vi "Robot Control.vi"() -> ()   [LabVIEW 2022 SP3]
uses:
  <vilib>/ImagingLab/Denso Robotics Library/_Private/Controls/drl_Motion parameters.ctl
  <vilib>/ImagingLab/Denso Robotics Library/_Private/Controls/drl_Interpolation.ctl
  <vilib>/ImagingLab/Denso Robotics Library/_Private/Controls/drl_Pass motion.ctl
  <vilib>/ImagingLab/Denso Robotics Library/_Private/Controls/drl_Move option.ctl
  <vilib>/ImagingLab/Denso Robotics Library/_Private/Controls/drl_Robot Coordinates.ctl
  <vilib>/ImagingLab/Denso Robotics Library/_Private/Controls/drl_Variable J.ctl
  <vilib>/ImagingLab/Denso Robotics Library/_Private/Controls/drl_Variable T.ctl
  <vilib>/ImagingLab/Denso Robotics Library/_Private/Controls/drl_TOOL.ctl
  <vilib>/ImagingLab/Denso Robotics Library/_Private/Controls/drl_arch_parameters.ctl
  <vilib>/ImagingLab/Denso Robotics Library/_Private/Controls/drl_Position Type.ctl
  <vilib>/ImagingLab/Denso Robotics Library/_Private/Controls/drl_Open Data.ctl
  <vilib>/ImagingLab/Denso Robotics Library/_Private/Controls/drl_Controller_IP Address.ctl
  <vilib>/ImagingLab/Denso Robotics Library/_Private/Controls/drl_Robot type.ctl
  <vilib>/ImagingLab/Denso Robotics Library/_Private/Controls/drl_controller_type.ctl
  <vilib>/ImagingLab/Denso Robotics Library/_Private/Controls/drl_Robot Session.ctl
  <vilib>/ImagingLab/Denso Robotics Library/_Private/Controls/drl_RobSlave actions.ctl
  <vilib>/ImagingLab/Denso Robotics Library/_Private/Controls/drl_Robot Motor status.ctl
  <vilib>/ImagingLab/Denso Robotics Library/_Private/Controls/drl_Get_Set.ctl
  <vilib>/Utility/error.llb/DialogType.ctl
  <vilib>/ImagingLab/Denso Robotics Library/_Public/SubVIs/drl_Get_Robot Position_P.vi
  <vilib>/ImagingLab/Denso Robotics Library/_Public/SubVIs/drl_Get_Robot Angle_J.vi
  <vilib>/ImagingLab/Denso Robotics Library/_Public/SubVIs/drl_Get_Robot Trans_T.vi
  <vilib>/ImagingLab/Denso Robotics Library/_Public/SubVIs/drl_Robot Move_CARTESIAN.vi
  <vilib>/ImagingLab/Denso Robotics Library/_Public/SubVIs/drl_Robot Move_JOINT.vi
  <vilib>/ImagingLab/Denso Robotics Library/_Public/SubVIs/drl_Set_Get Variable_P.vi
  <vilib>/ImagingLab/Denso Robotics Library/DensoRoboticsLibrary.lvlib
panel:
  in  "Main Tab Control":T1(tab)
  in  "Move Tab Control":enum32{"Cartesian", "Joint"}(tab)
  in  "Move to position C":bool
  in  "robot coordinates C":T2 {"X" format="%.4f"; "Y" format="%.4f"; "Z" format="%.4f"; "Rx" format="%.4f"; "Ry" format="%.4f"; "Rz" format="%.4f"}
  in  "motion parameters C":T3
  in  "Load position C":bool
  in  "Move to position J":bool
  in  "motion parameters J":T3
  in  "Load position J":bool
  in  "robot coordinates J":T7 {"Axis 6" format="%.4f"; "Axis 5" format="%.4f"; "Axis 4" format="%.4f"; "Axis 3" format="%.4f"; "Axis 2" format="%.4f"; "Axis 1" format="%.4f"}
  in  "Set tool active":bool
  in  "Set tool params":bool
  in  "Tool data":T8
  in  "Tool number set":i32
  in  "Active tool":i32
  in  "Tab Control":enum32{"Cart", "Joint"}(tab)
  in  "Drive cart":bool
  out "Velocity start cart":T2 {"X" format="%.4f"; "Y" format="%.4f"; "Z" format="%.4f"; "Rx" format="%.4f"; "Ry" format="%.4f"; "Rz" format="%.4f"}
  out "Current step cart":i32
  in  "velocity motion parameters cart":T3
  in  "Velocity step cart":T2 {"X" format="%.4f"; "Y" format="%.4f"; "Z" format="%.4f"; "Rx" format="%.4f"; "Ry" format="%.4f"; "Rz" format="%.4f"}
  in  "Steps cart":i32
  in  "Drive joint":bool
  out "Velocity start joint":T7 {"Axis 6" format="%.4f"; "Axis 5" format="%.4f"; "Axis 4" format="%.4f"; "Axis 3" format="%.4f"; "Axis 2" format="%.4f"; "Axis 1" format="%.4f"}
  in  "velocity motion parameters joint":T3
  out "Current step joint":i32
  in  "Velocity step joint":T7 {"Axis 6" format="%.4f"; "Axis 5" format="%.4f"; "Axis 4" format="%.4f"; "Axis 3" format="%.4f"; "Axis 2" format="%.4f"; "Axis 1" format="%.4f"}
  in  "Steps joints":i32
  in  "Start arch":bool
  in  "position type":T9
  in  "variable P end":T2 {"X" format="%.4f"; "Y" format="%.4f"; "Z" format="%.4f"; "Rx" format="%.4f"; "Ry" format="%.4f"; "Rz" format="%.4f"}
  in  "arch parameters":T10={"height (mm)"=5, "arch start (mm)"=0, "arch finish (mm)"=0}
  in  "Internal speed":dbl=100.0
  in  "External speed":dbl=10.0
  in  "stop":bool
  out "position T":T11 {"Az" format="%.4f"; "Ay" format="%.4f"; "Ax" format="%.4f"; "Oz" format="%.4f"; "Oy" format="%.4f"; "Ox" format="%.4f"; "Z" format="%.4f"; "Y" format="%.4f"; "X" format="%.4f"}
  out "position J":T7 {"Axis 6" format="%.4f"; "Axis 5" format="%.4f"; "Axis 4" format="%.4f"; "Axis 3" format="%.4f"; "Axis 2" format="%.4f"; "Axis 1" format="%.4f"}
  out "position P":T2 {"X" format="%.4f"; "Y" format="%.4f"; "Z" format="%.4f"; "Rx" format="%.4f"; "Ry" format="%.4f"; "Rz" format="%.4f"}
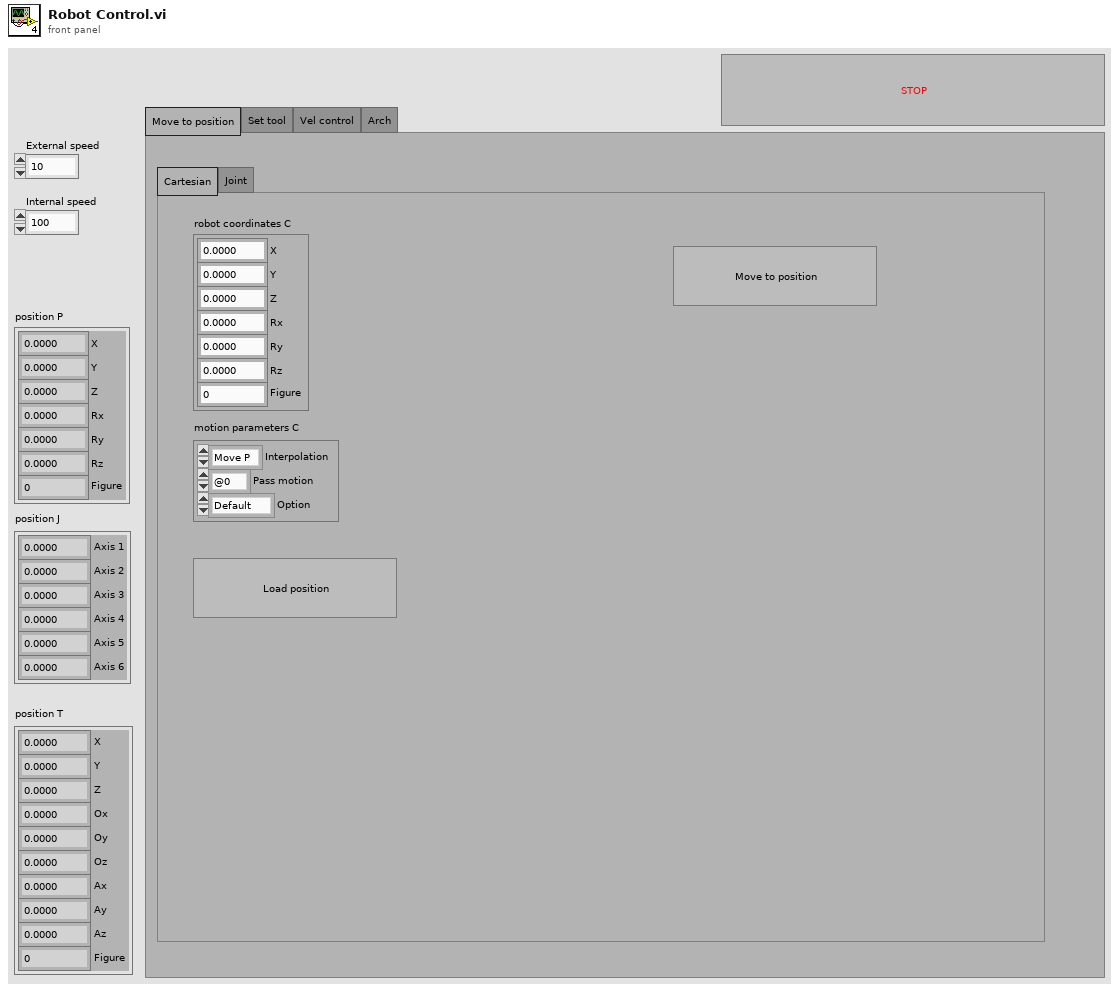
[diagram p1: front panel]
types:
  T1 = enum32{"Move to position", "Set tool", "Vel control", "Arch"}
  T2 = typedef "DensoRoboticsLibrary.lvlib/drl_Robot Coordinates.ctl" = cluster{"X":dbl, "Y":dbl, "Z":dbl, "Rx":dbl, "Ry":dbl, "Rz":dbl, "Figure":dbl}
  T3 = typedef "DensoRoboticsLibrary.lvlib/drl_Motion parameters.ctl" = cluster{"Interpolation":T4, "Pass motion":T5, "Option":T6}
  T4 = typedef "DensoRoboticsLibrary.lvlib/drl_Interpolation.ctl" = enum16{"Move P", "Move L"}
  T5 = typedef "DensoRoboticsLibrary.lvlib/drl_Pass motion.ctl" = enum16{"@0", "@P", "@E"}
  T6 = typedef "DensoRoboticsLibrary.lvlib/drl_Move option.ctl" = enum16{"Default", "Next"}
  T7 = typedef "DensoRoboticsLibrary.lvlib/drl_Variable J.ctl" = cluster{"Axis 1":sgl, "Axis 2":sgl, "Axis 3":sgl, "Axis 4":sgl, "Axis 5":sgl, "Axis 6":sgl}
  T8 = typedef "DensoRoboticsLibrary.lvlib/drl_TOOL.ctl" = cluster{"X":sgl, "Y":sgl, "Z":sgl, "RX":sgl, "RY":sgl, "RZ":sgl}
  T9 = typedef "DensoRoboticsLibrary.lvlib/drl_Position Type.ctl" = enum16{"P", "J", "T"}
  T10 = typedef "DensoRoboticsLibrary.lvlib/drl_arch_parameters.ctl" = cluster{"height (mm)":i32, "arch start (mm)":i32, "arch finish (mm)":i32}
  T11 = typedef "DensoRoboticsLibrary.lvlib/drl_Variable T.ctl" = cluster{"X":sgl, "Y":sgl, "Z":sgl, "Ox":sgl, "Oy":sgl, "Oz":sgl, "Ax":sgl, "Ay":sgl, "Az":sgl, "Figure":sgl}
  T12 = typedef "DensoRoboticsLibrary.lvlib/drl_RobSlave actions.ctl" = enum16{"Start", "Stop"}
  T13 = typedef "DensoRoboticsLibrary.lvlib/drl_Robot Motor status.ctl" = enum16{"Motor OFF", "Motor ON"}
  T14 = typedef "DensoRoboticsLibrary.lvlib/drl_Robot Session.ctl" = string
  T15 = typedef "DensoRoboticsLibrary.lvlib/drl_Open Data.ctl" = cluster{"controller IP address":T16, "robot type":T17, "controller type":T18}
  T16 = typedef "DensoRoboticsLibrary.lvlib/drl_Controller_IP Address.ctl" = string
  T17 = typedef "DensoRoboticsLibrary.lvlib/drl_Robot type.ctl" = enum16{"6 axes", "5 axes", "4 axes"}
  T18 = typedef "DensoRoboticsLibrary.lvlib/drl_controller_type.ctl" = enum16{"RC7", "RC8"}
  T19 = typedef "DensoRoboticsLibrary.lvlib/drl_Get_Set.ctl" = enum16{"Get", "Set"}
  T20 = typedef "DialogType.ctl" = u16
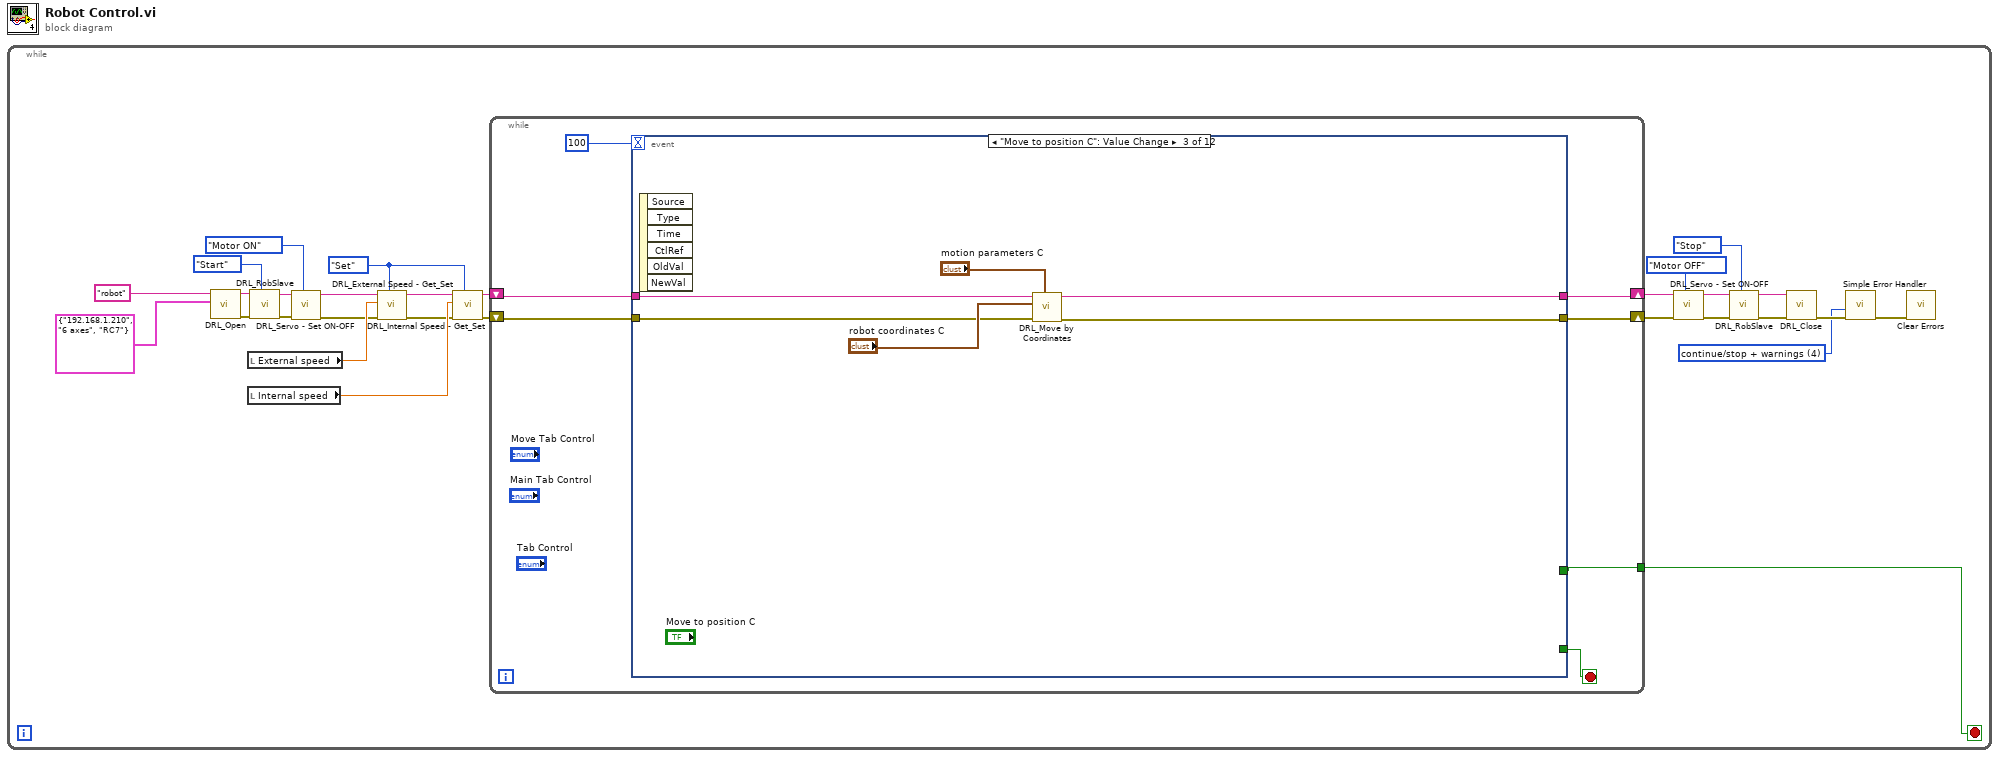
[diagram p0: block diagram]
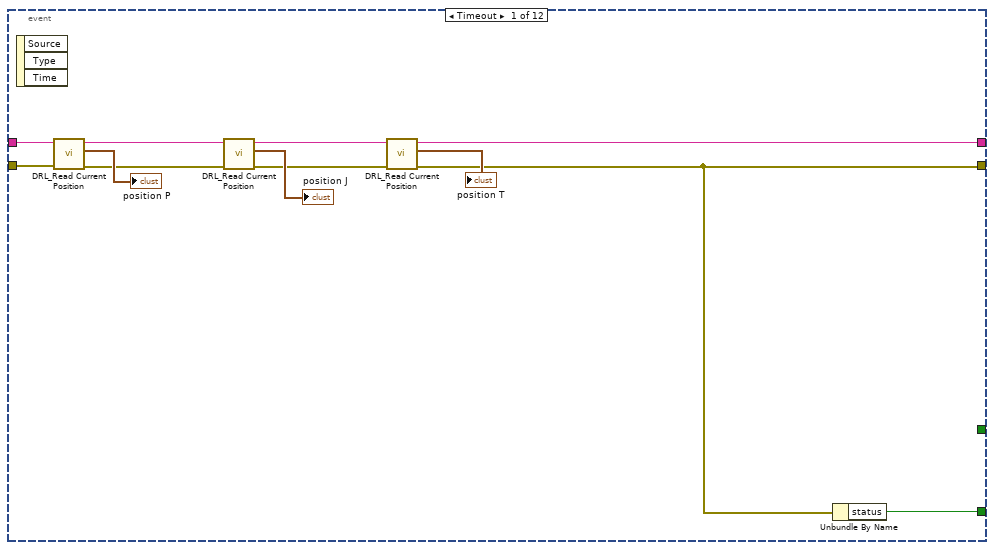
[diagram p2: hidden frame]
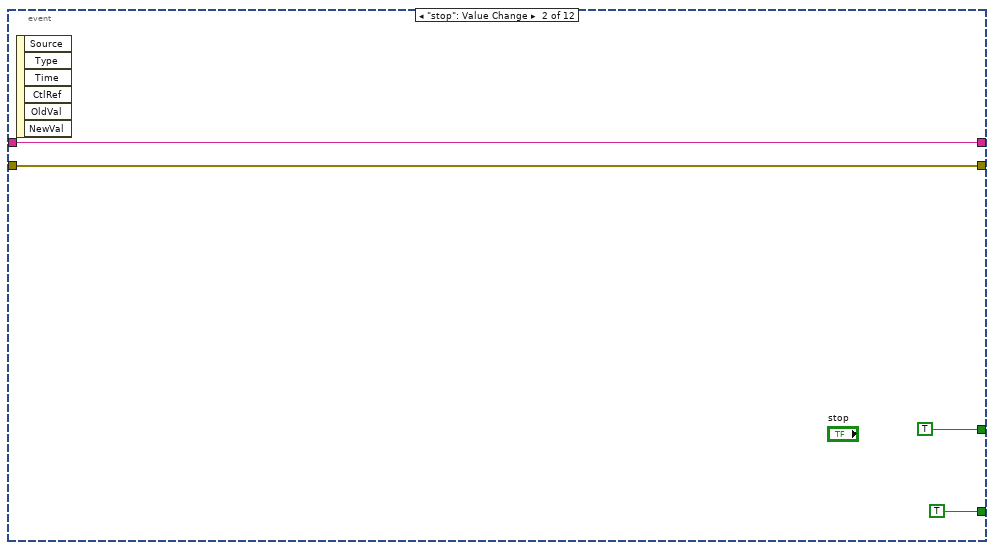
[diagram p3: hidden frame]
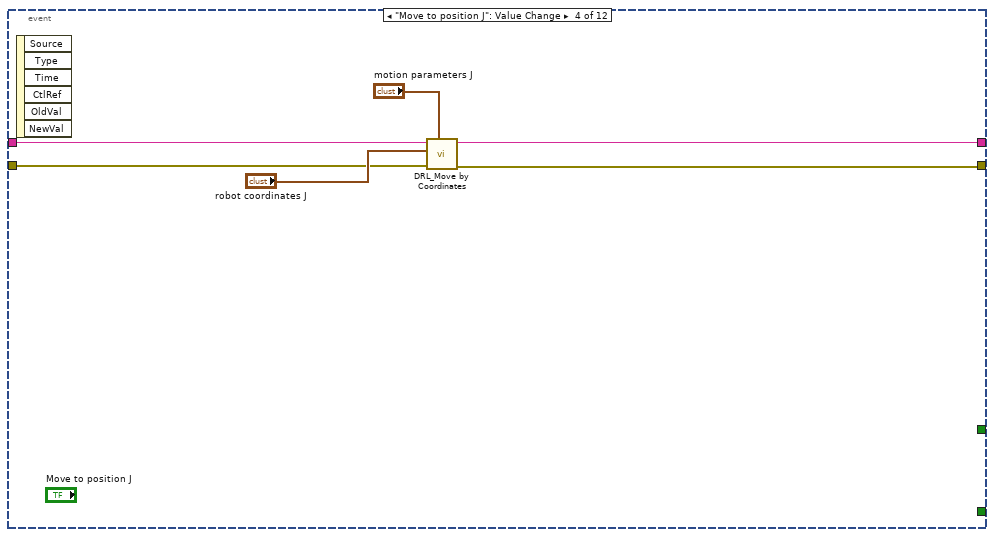
[diagram p4: hidden frame]
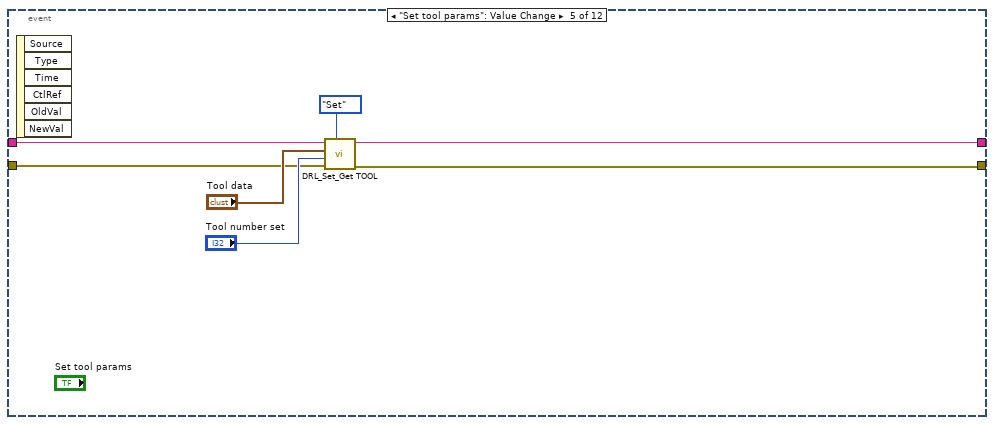
[diagram p5: hidden frame]
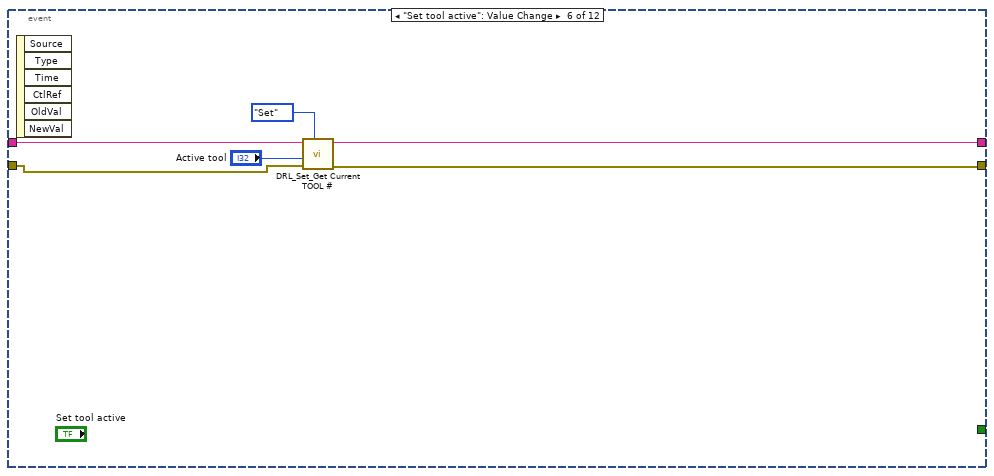
[diagram p6: hidden frame]
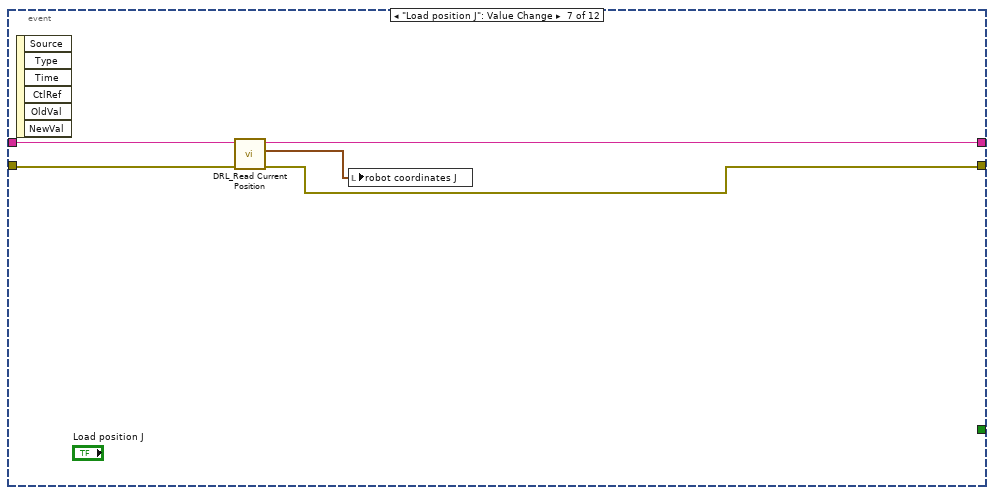
[diagram p7: hidden frame]
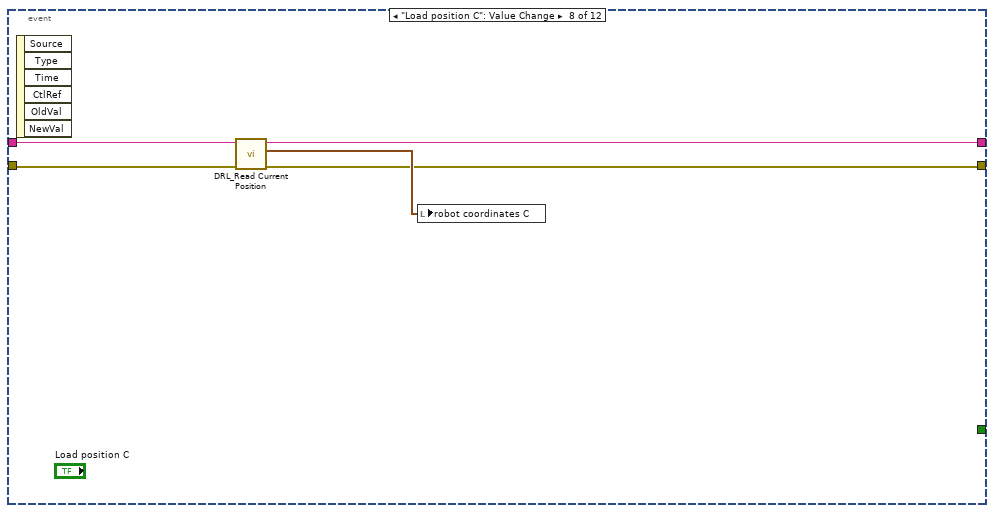
[diagram p8: hidden frame]
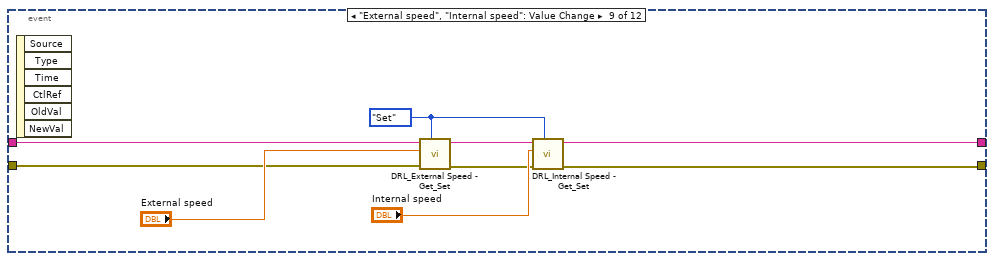
[diagram p9: hidden frame]
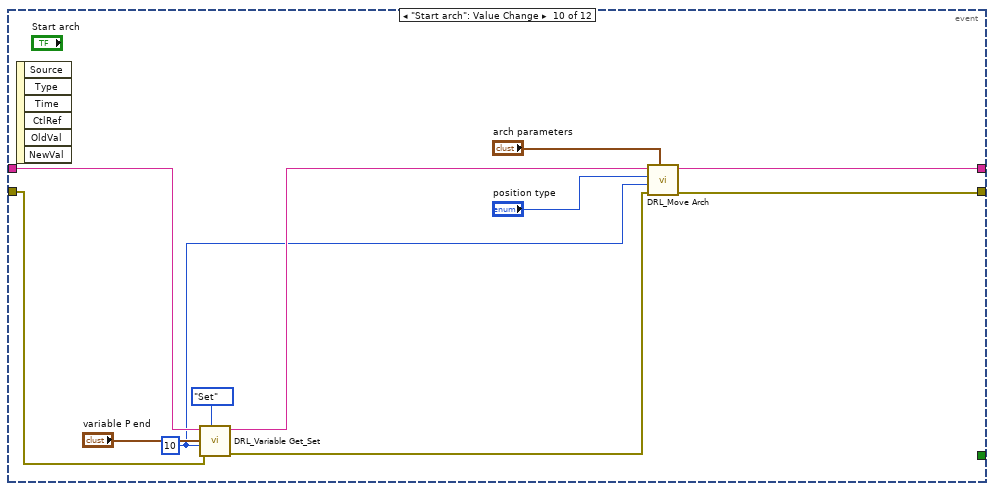
[diagram p10: hidden frame]
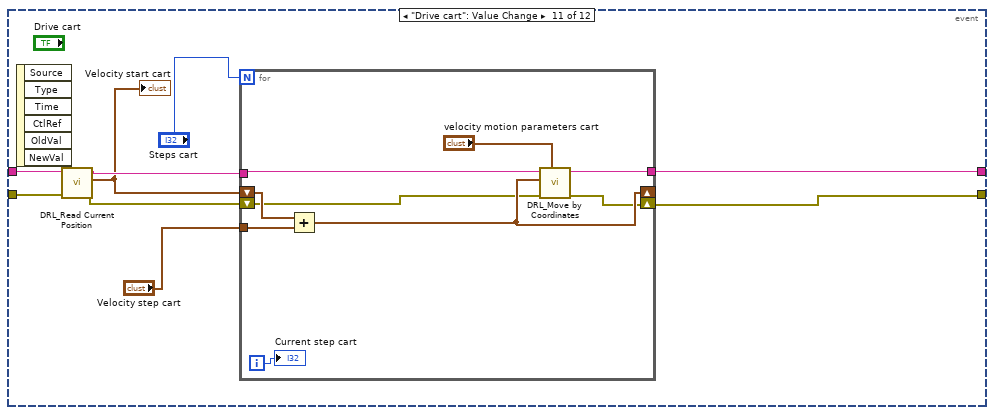
[diagram p11: hidden frame]
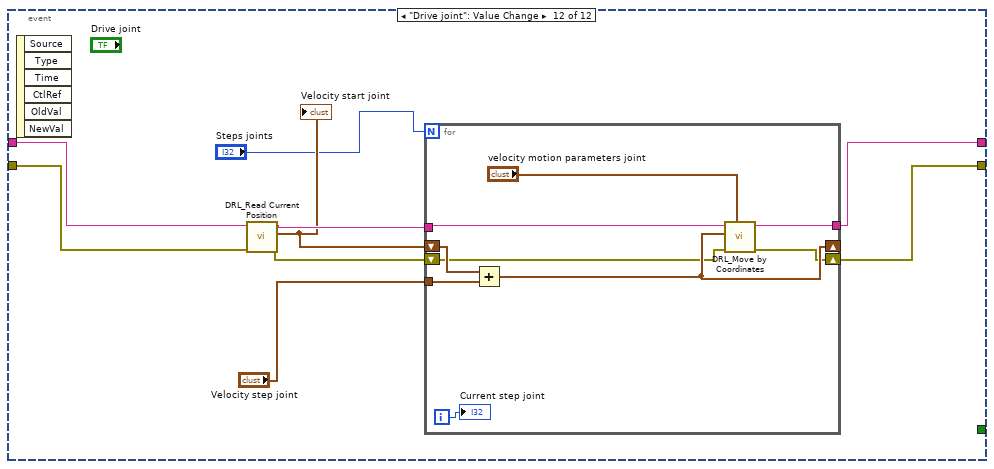
[diagram p12: hidden frame]
diagram:
  n1 = while {
    stop <- w1 stop-if-true
    w3 = T20 4 items=["no dialog", "OK message", "continue or stop message", "OK message + warnings", "continue/stop + warnings"] ("type of dialog (OK msg:1)")
    w13 = drl_Get_Set."Set" ("action")
    n2 = call <vilib>:"DRL_Open.vi"("connection settings"=T15 {"controller IP address"="192.168.1.210", "robot type"=enum."6 axes", "controller type"=enum."RC7"}, "robot session"=T14 "robot") -> ("error out"=w12:errorcluster, "robot session*"=w27:T14)  [unwired: 8 in]
    n3 = local read "External speed"() -> (w15:dbl)
    n4 = local read "Internal speed"() -> (w14:dbl)
    n5 = call <vilib>:"DRL_RobSlave.vi"("action"=drl_RobSlave_actions."Start", "error in (no error)"=w12, "robot session"=w27) -> ("error out"=w11:errorcluster, "robot session*"=w26:T14)  [unwired: 7 in]
    n6 = call <vilib>:"DRL_Servo - Set ON-OFF.vi"("servo status"=drl_Robot_Motor_status."Motor ON", "error in (no error)"=w11, "robot session"=w26) -> ("error out"=w10:errorcluster, "robot session*"=w17:T14)  [unwired: 7 in]
    n7 = call <vilib>:"DRL_External Speed - Get_Set.vi"("action"=w13, "error in (no error)"=w10, "ext speed in"=w15, "robot session"=w17) -> ("error out"=w9:errorcluster, "robot session*"=w18:T14)  [unwired: 5 in, 1 out]
    n8 = call <vilib>:"DRL_Internal Speed - Get_Set.vi"("action"=w13, "error in (no error)"=w9, "int speed in"=w14, "robot session"=w18) -> ("error out"=w8:errorcluster, "robot session*"=w16:T14)  [unwired: 5 in, 1 out]
    n9 = while {
      shift-right: [w35] -> w23
      shift-left: w16 -> [w36]
      shift-right: [w31] -> w7
      shift-left: w8 -> [w32]
      tunnel: [w30] -> w1
      stop <- w33 stop-if-true
      n10 = event shown="[2] \"Move to position C\": Value Change" {
        selector: _ -> [_ _ _ _ _ _ _ _ _ _ _ _]
        dyn-events: _ -> [_ _ _ _ _ _ _ _ _ _ _ _]
        timeout: 100 -> [_ _ _ _ _ _ _ _ _ _ _ _]
        tunnel: w36 -> [w48 w52 w58 w64 w70 w77 w82 w87 w96 w102 w116 w132]
        tunnel: [w44 w52 w55 w63 w67 w76 w81 w86 w94 w107 w115 w130] -> w35
        tunnel: [w37 TRUE _ _ _ _ _ _ _ _ _ _] -> w33
        tunnel: w32 -> [w41 w50 w54 w60 w66 w73 w79 w84 w90 w99 w110 w128]
        tunnel: [w38 w50 w53 w59 w65 w72 w78 w83 w88 w97 w108 w126] -> w31
        tunnel: [_ TRUE _ _ _ _ _ _ _ _ _ _] -> w30
        event Timeout {
          n11 = event-data() -> ()  [unwired: 1 in, 3 out]
          n12 = call-poly <vilib>:"DRL_Read Current Position.vi"("error in (no error)"=w41, "robot session"=w48) -> ("error out"=w40:errorcluster, "position P"=→"position P":T2, "robot session*"=w46:T14)  [unwired: 7 in]
          n13 = call-poly <vilib>:"DRL_Read Current Position.vi"("error in (no error)"=w40, "robot session"=w46) -> ("error out"=w39:errorcluster, "position J"=→"position J":T7, "robot session*"=w45:T14)  [unwired: 7 in]
          n14 = call-poly <vilib>:"DRL_Read Current Position.vi"("error in (no error)"=w39, "robot session"=w45) -> ("error out"=w38:errorcluster, "position T"=→"position T":T11, "robot session*"=w44:T14)  [unwired: 7 in]
          n15 = Unbundle By Name(w38) -> ("status"=w37:bool)
        }
        event "stop": Value Change {
          n16 = event-data() -> ()  [unwired: 1 in, 6 out]
        }
        event "Move to position C": Value Change {
          n17 = event-data() -> ()  [unwired: 1 in, 6 out]
          n18 = call-poly <vilib>:"DRL_Move by Coordinates.vi"("motion parameters"="motion parameters C", "error in (no error)"=w54, "robot coordinates"="robot coordinates C", "robot session"=w58) -> ("error out"=w53:errorcluster, "robot session*"=w55:T14)  [unwired: 6 in]
        }
        event "Move to position J": Value Change {
          n19 = event-data() -> ()  [unwired: 1 in, 6 out]
          n20 = call-poly <vilib>:"DRL_Move by Coordinates.vi"("motion parameters"="motion parameters J", "error in (no error)"=w60, "position J"="robot coordinates J", "robot session"=w64) -> ("error out"=w59:errorcluster, "robot session*"=w63:T14)  [unwired: 6 in]
        }
        event "Set tool params": Value Change {
          n21 = event-data() -> ()  [unwired: 1 in, 6 out]
          n22 = call <vilib>:"DRL_Set_Get TOOL.vi"("action"=drl_Get_Set."Set", "error in (no error)"=w66, "tool number"="Tool number set", "tool data in"="Tool data", "robot session"=w70) -> ("error out"=w65:errorcluster, "robot session*"=w67:T14)  [unwired: 4 in, 1 out]
        }
        event "Set tool active": Value Change {
          n23 = event-data() -> ()  [unwired: 1 in, 6 out]
          n24 = call <vilib>:"DRL_Set_Get Current TOOL #.vi"("action"=drl_Get_Set."Set", "error in (no error)"=w73, "ID number in"="Active tool", "robot session"=w77) -> ("error out"=w72:errorcluster, "robot session"=w76:T14)  [unwired: 5 in, 1 out]
        }
        event "Load position J": Value Change {
          n25 = event-data() -> ()  [unwired: 1 in, 6 out]
          n26 = call-poly <vilib>:"DRL_Read Current Position.vi"("error in (no error)"=w79, "robot session"=w82) -> ("error out"=w78:errorcluster, "position J"=w80:T7, "robot session*"=w81:T14)  [unwired: 7 in]
          n27 = local write "robot coordinates J"(w80) -> ()
        }
        event "Load position C": Value Change {
          n28 = event-data() -> ()  [unwired: 1 in, 6 out]
          n29 = call-poly <vilib>:"DRL_Read Current Position.vi"("error in (no error)"=w84, "robot session"=w87) -> ("error out"=w83:errorcluster, "position P"=w85:T2, "robot session*"=w86:T14)  [unwired: 7 in]
          n30 = local write "robot coordinates C"(w85) -> ()
        }
        event "External speed", "Internal speed": Value Change {
          w91 = drl_Get_Set."Set" ("action")
          n31 = event-data() -> ()  [unwired: 1 in, 6 out]
          n32 = call <vilib>:"DRL_External Speed - Get_Set.vi"("action"=w91, "error in (no error)"=w90, "ext speed in"="External speed", "robot session"=w96) -> ("error out"=w89:errorcluster, "robot session*"=w95:T14)  [unwired: 5 in, 1 out]
          n33 = call <vilib>:"DRL_Internal Speed - Get_Set.vi"("action"=w91, "error in (no error)"=w89, "int speed in"="Internal speed", "robot session"=w95) -> ("error out"=w88:errorcluster, "robot session*"=w94:T14)  [unwired: 5 in, 1 out]
        }
        event "Start arch": Value Change {
          w100 = 10 ("variable number")
          n34 = event-data() -> ()  [unwired: 1 in, 6 out]
          n35 = call-poly <vilib>:"DRL_Variable Get_Set.vi"("action"=drl_Get_Set."Set", "error in (no error)"=w99, "variable number"=w100, "variable P in"="variable P end", "robot session"=w102) -> ("error out"=w98:errorcluster, "robot session*"=w103:T14)  [unwired: 4 in, 1 out]
          n36 = call <vilib>:"DRL_Move Arch.vi"("arch parameters"="arch parameters", "error in (no error)"=w98, "position number"=w100, "position type"="position type", "robot session"=w103) -> ("error out"=w97:errorcluster, "robot session*"=w107:T14)  [unwired: 5 in]
        }
        event "Drive cart": Value Change {
          n37 = event-data() -> ()  [unwired: 1 in, 6 out]
          n38 = call-poly <vilib>:"DRL_Read Current Position.vi"("error in (no error)"=w110, "robot session"=w116) -> ("error out"=w109:errorcluster, "position P"=w112:T2, "robot session*"=w113:T14)  [unwired: 7 in]
          "Velocity start cart" <- w112
          n39 = for {
            N: "Steps cart" -> [_]
            tunnel: [w125] -> w115
            tunnel: w113 -> [w122]
            shift-right: [w120] -> _
            shift-left: w112 -> [w124]
            tunnel: "Velocity step cart" -> [w123]
            shift-right: [w117] -> w108
            shift-left: w109 -> [w118]
            i -> [w119]
            n40 = Add(x=w124, y=w123) -> (x+y=w120:T2)
            n41 = call-poly <vilib>:"DRL_Move by Coordinates.vi"("motion parameters"="velocity motion parameters cart", "error in (no error)"=w118, "robot coordinates"=w120, "robot session"=w122) -> ("error out"=w117:errorcluster, "robot session*"=w125:T14)  [unwired: 6 in]
            "Current step cart" <- w119
          }
        }
        event "Drive joint": Value Change {
          n42 = event-data() -> ()  [unwired: 1 in, 6 out]
          n43 = call-poly <vilib>:"DRL_Read Current Position.vi"("error in (no error)"=w128, "robot session"=w132) -> ("error out"=w127:errorcluster, "position J"=w133:T7, "robot session*"=w134:T14)  [unwired: 7 in]
          "Velocity start joint" <- w133
          n44 = for {
            N: "Steps joints" -> [_]
            tunnel: [w143] -> w130
            tunnel: w134 -> [w141]
            shift-right: [w139] -> _
            shift-left: w133 -> [w142]
            tunnel: "Velocity step joint" -> [w137]
            shift-right: [w135] -> w126
            shift-left: w127 -> [w136]
            i -> [w138]
            n45 = Add(x=w142, y=w137) -> (x+y=w139:T7)
            n46 = call-poly <vilib>:"DRL_Move by Coordinates.vi"("motion parameters"="velocity motion parameters joint", "error in (no error)"=w136, "position J"=w139, "robot session"=w141) -> ("error out"=w135:errorcluster, "robot session*"=w143:T14)  [unwired: 6 in]
            "Current step joint" <- w138
          }
        }
      }
    }
    n47 = call <vilib>:"DRL_Servo - Set ON-OFF.vi"("servo status"=drl_Robot_Motor_status."Motor OFF", "error in (no error)"=w7, "robot session"=w23) -> ("error out"=w6:errorcluster, "robot session*"=w22:T14)  [unwired: 7 in]
    n48 = call <vilib>:"DRL_RobSlave.vi"("action"=drl_RobSlave_actions."Stop", "error in (no error)"=w6, "robot session"=w22) -> ("error out"=w5:errorcluster, "robot session*"=w21:T14)  [unwired: 7 in]
    n49 = call <vilib>:"DRL_Close.vi"("error in (no error)"=w5, "robot session"=w21) -> ("error out"=w4:errorcluster)  [unwired: 9 in]
    n50 = call <vilib>:"Simple Error Handler.vi"("type of dialog (OK msg:1)"=w3, "error in (no error)"=w4) -> ("error out"=w2:errorcluster)  [unwired: 3 in, 4 out]
    n51 = call <vilib>:"Clear Errors.vi"("error in (no error)"=w2) -> ()  [unwired: 5 in, 2 out]
  }
